vi "EventLogger.Init.TMOS.vi"(8 "error in":errorcluster, 10 "Description":string="TMOS log") -> (0 "error out":errorcluster, 3 "EventLog ref out":refnum<class "EventLog.lvclass">)   [LabVIEW 2019, in "Tools.lvlib"]
uses:
  Tools.lvlib
  <vilib>/NI/Event Logger Library/EventLog/EventLog.lvclass
  <vilib>/NI/Event Logger Library/EventBuffer/Options.ctl
  <vilib>/NI/Event Logger Library/EventBuffer/EventBuffer.lvclass
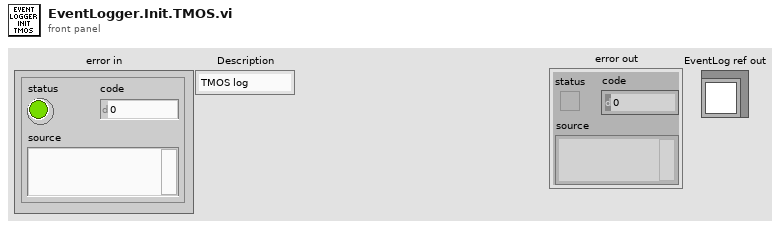
[diagram p1: front panel]
types:
  T1 = enum16{"Settings dir", "Logs dir", "Resources dir", "Verification file", "Users file", "Root dir"}
  T2 = typedef "EventBuffer.lvclass/Options.ctl" = cluster{"Max elements":dbl, "Max string length":dbl}
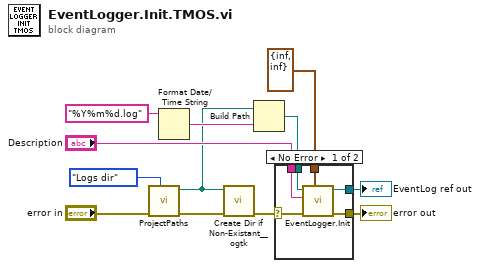
[diagram p0: block diagram]
diagram:
  n1 = call "ProjectPaths.vi"("Item"=T1."Logs dir", "Error In"="error in") -> ("Error Out"=w2:errorcluster, "Path"=w3:path)  [unwired: 8 in]
  n2 = Format Date/Time String(time format string (%c)="%Y%m%d.log") -> (date/time string=w11:string)  [unwired: 2 in]
  n3 = call <userlib>:"Create Dir if Non-Existant__ogtk.vi"("error in (no error)"=w2, "Directory Path"=w3) -> ("error out"=w5:errorcluster)  [unwired: 7 in, 2 out]
  n4 = Build Path(base path=w3, name or relative path=w11) -> (appended path=w10:path)
  n5 = case shown="No Error" w5 {
    selector: w5 -> [w13 w19]
    tunnel: w10 -> [w18 _]
    tunnel: [w17 w19] -> w9
    tunnel: "Description" -> [w16 _]
    tunnel: [w15 _] -> w7
    tunnel: T2 {"Max elements"=inf, "Max string length"=inf} ("Options") -> [w14 _]
    frame No Error {
      n6 = call "EventLogger.Init.vi"("Options"=w14, "error in"=w13, "Description"=w16, "Path"=w18) -> ("error out"=w17:errorcluster, "EventLog ref out"=w15:refnum<class "EventLog.lvclass">)  [unwired: 6 in]
    }
    frame Error {
    }
  }
  "error out" <- w9
  "EventLog ref out" <- w7
